vi "Try Read Discovery UDP.vi"(8 "error in (no error)":errorcluster, 11 "DiscoveryService in":refnum<class "DiscoveryService.lvclass">) -> (0 "error out":errorcluster, 3 "DiscoveryService out":refnum<class "DiscoveryService.lvclass">)   [LabVIEW 2020, in "Vecto.lvlib" / "DiscoveryService.lvclass"]
uses:
  DiscoveryService.lvclass
  DiscoveryService.lvclass/DiscoveryService.ctl
  <vilib>/Utility/error.llb/Error Cluster From Error Code.vi
  Vecto.lvlib
  lv-volatus/messages/Discovery/Discovery.lvlib
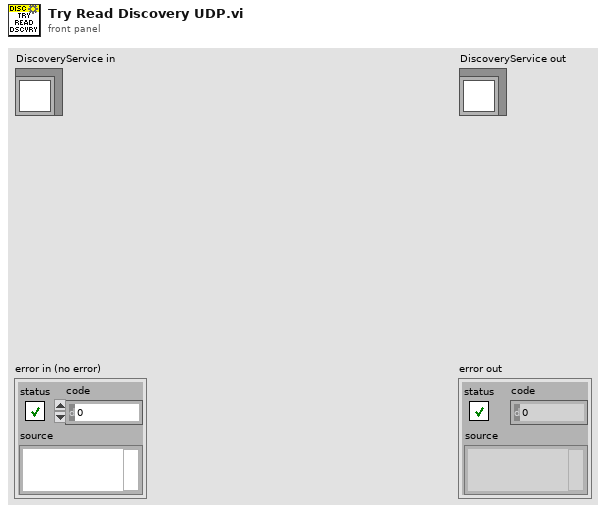
[diagram p1: front panel]
types:
  T1 = typedef "UdpPayload.lvlib/Data.ctl" = cluster{"source_id":u32, "sequence":u32, "timestamp":i64, "type":string, "payload":u8[]}
  T2 = typedef "Discovery.lvlib/Data.ctl" = cluster{"node_id":u32, "name":string, "ip":u32, "status":string, "services":T3[], "capabilities":string[], "system":string, "cluster":string, "app_version":string, "cfg_version":string}
  T3 = typedef "Service.lvlib/Data.ctl" = cluster{"type":T4, "port":i32}
  T4 = typedef "ServiceType.lvlib/Enumeration.ctl" = enum16{"SERVICETYPE_UNKNOWN", "SERVICETYPE_TCPSERVER", "SERVICETYPE_HTTPSERVER"}
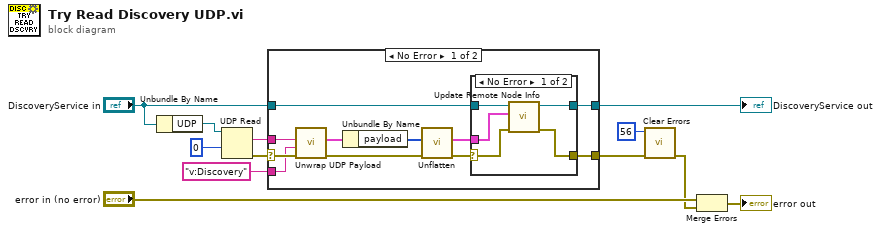
[diagram p0: block diagram]
diagram:
  n1 = Unbundle By Name("DiscoveryService in") -> ("UDP"=w11:refnum<k16>)
  n2 = UDP Read(connection ID=w11, timeout ms (25000)=0) -> (data out=w3:string, error out=w2:errorcluster)  [unwired: 2 in, 3 out]
  n3 = case shown="No Error" w2 {
    selector: w2 -> [w19 w32]
    tunnel: "DiscoveryService in" -> [w23 w31]
    tunnel: [w22 w32] -> w8
    tunnel: [w21 w31] -> w4
    tunnel: w3 -> [w20 _]
    tunnel: "v:Discovery" ("Discovery") -> [w18 _]
    frame No Error {
      n4 = call "Unwrap UDP Payload.vi"("error in (no error)"=w19, "Expected Type (Any)"=w18, "UDP Payload"=w20) -> ("error out"=w15:errorcluster, "Data"=w17:T1)  [unwired: 7 in]
      n5 = Unbundle By Name(w17) -> ("payload"=w16:u8[])
      n6 = call "Unflatten.vi"("error in"=w15, "Buffer"=w16) -> ("error out"=w13:errorcluster, "Data"=w14:T2)  [unwired: 8 in]
      n7 = case shown="No Error" w13 {
        selector: w13 -> [w24 w29]
        tunnel: w23 -> [w28 w30]
        tunnel: [w27 w29] -> w22
        tunnel: [w26 w30] -> w21
        tunnel: w14 -> [w25 _]
        frame No Error {
          n8 = call "Update Remote Node Info.vi"("error in (no error)"=w24, "Discovery"=w25, "DiscoveryService in"=w28) -> ("error out"=w27:errorcluster, "DiscoveryService out"=w26:refnum<class "DiscoveryService.lvclass">)  [unwired: 7 in]
        }
        frame Error {
        }
      }
    }
    frame Error {
    }
  }
  "DiscoveryService out" <- w4
  n9 = call <vilib>:"Clear Errors.vi"("error in (no error)"=w8, "specific error code to clear (0: all)"=56) -> ("error out"=w5:errorcluster)  [unwired: 4 in, 1 out]
  n10 = Merge Errors("error in (no error)", w5) -> (→"error out":errorcluster)
